vi "insert values.vi"(5 "是否创建唯一键":bool, 7 "data":variant[](array[variant]), 8 "错误输入（无错误）":errorcluster, 9 "columns外部输入":T1, 10 "database":string="database1", 11 "Tabe Name":string) -> (0 "错误输出":errorcluster)   [LabVIEW 2016]
uses:
  Access/Access Lib.lvlib
  SQLite/SQLite Lib.lvlib
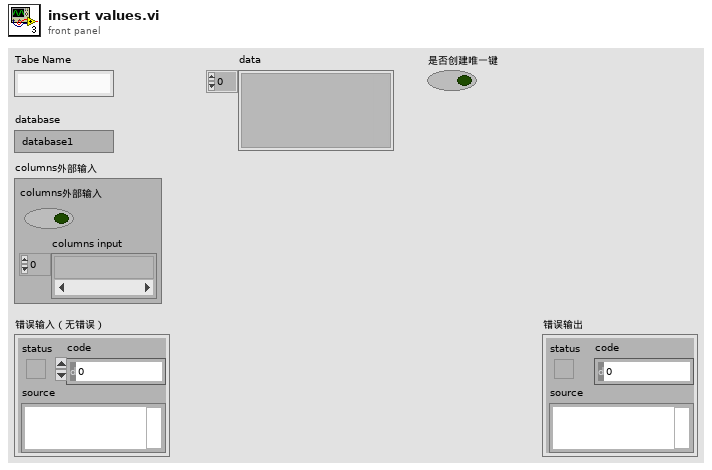
[diagram p1: front panel]
types:
  T1 = cluster{"columns外部输入":bool, "columns input":string[]}
  T2 = typedef "数据库类型.ctl" = enum16{"Access", "SQLite"}
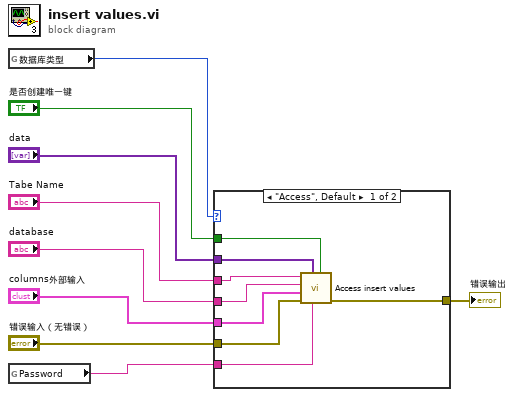
[diagram p0: block diagram]
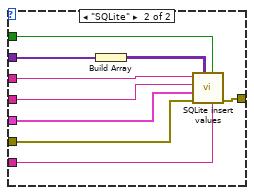
[diagram p2: hidden frame]
diagram:
  n1 = global read "外部调用接口全局变量.vi" "数据库类型"() -> (w1:T2)
  n2 = global read "外部调用接口全局变量.vi" "Password"() -> (w2:string)
  n3 = case shown="\"Access\", Default" w1 {
    tunnel: "Tabe Name" -> [w13 w26]
    tunnel: "是否创建唯一键" -> [w16 w25]
    tunnel: "错误输入（无错误）" -> [w15 w24]
    tunnel: [w14 w23] -> w6
    tunnel: "data" -> [w17 w22]
    tunnel: "database" -> [w12 w20]
    tunnel: "columns外部输入" -> [w11 w19]
    tunnel: w2 -> [w10 w18]
    frame "Access", Default {
      n4 = call "Access insert values.vi"("是否创建唯一键"=w16, "Password"=w10, "data"=w17, "error in (no error)"=w15, "columns外部输入"=w11, "database"=w12, "table"=w13) -> ("error out"=w14:errorcluster)  [unwired: 4 in]
    }
    frame "SQLite" {
      n5 = Build Array(w22) -> (w21:variant[][])
      n6 = call "SQLite insert values.vi"("Password"=w18, "是否创建唯一键"=w25, "数组"=w21, "错误输入（无错误）"=w24, "columns外部输入"=w19, "database"=w20, "Tabe Name"=w26) -> ("错误输出"=w23:errorcluster)  [unwired: 4 in]
    }
  }
  "错误输出" <- w6
